vi "Current_Step.vi"   [LabVIEW 2019]
uses:
  Instrument_Setup.vi
  Global/Global Variables/Data_Display_global.vi
  Global/Global Variables/global.vi
  Equipment/Keithley 24XX/Keithley 24XX.lvlib
types:
  T1 = typedef "16T-Cluster.ctl" = cluster{"Clamp":bool, "Switch Heater":bool, "Go to Zero":bool, "Go to set":bool, "Go to Hold":bool, "Clamped":bool, "Quenched":bool, "Rate limit":bool, "Persistent":bool, "Hold":bool, "Set":bool, "Zero":bool, "Magnet (T)":dbl, "Leads (T)":dbl, "Magnet T (K)":dbl, "Switch":bool, "Setpoint (T)":dbl, "Rate (T/min)":dbl, "Select":bool, "Sweeping":bool}
  T2 = typedef "PSIO.ctl" = cluster{"Address":T3, "Version":enum16{"PS", "IPS"}}
  T3 = typedef "OxfordAddress.ctl" = cluster{"Com Port":i32, "ISOBUS Address":i32, "GPIB Address":i16, "Communication":enum16{"RS232", "ISOBUS", "GPIB", "Gateway"}}
  T4 = cluster{"Version\n":string, "Max Sweep(4.2K)":dbl[unit], "Max Sweep(2.2K)":dbl[unit], "Switch htr dly":dbl[unit], "Max Field(4.2K)":dbl[unit], "Max Field(2.2K)":dbl[unit], "Max lead res":dbl[unit], "IO Info":T2}
  T5 = typedef "15T-Cluster.ctl" = cluster{"Magnet (T)":dbl, "Leads (T)":dbl, "Setpoint (T)":dbl, "Rate (T/min)":dbl, "Set":bool, "Zero":bool, "Hold":bool, "Go to zero":bool, "Go to Hold":bool, "Go to Set":bool, "Clamp":bool, "Switch Heater":bool, "Rate limit":bool, "Switch":bool, "Clamped":bool, "Persistent":bool, "Quenched":bool, "Sweeping":bool, "Select":bool}
  T6 = cluster{"Version\n":string, "Max Sweep":dbl[unit], "Max Field":dbl[unit], "IO Info":T2, "Switch htr dly":dbl[unit]}
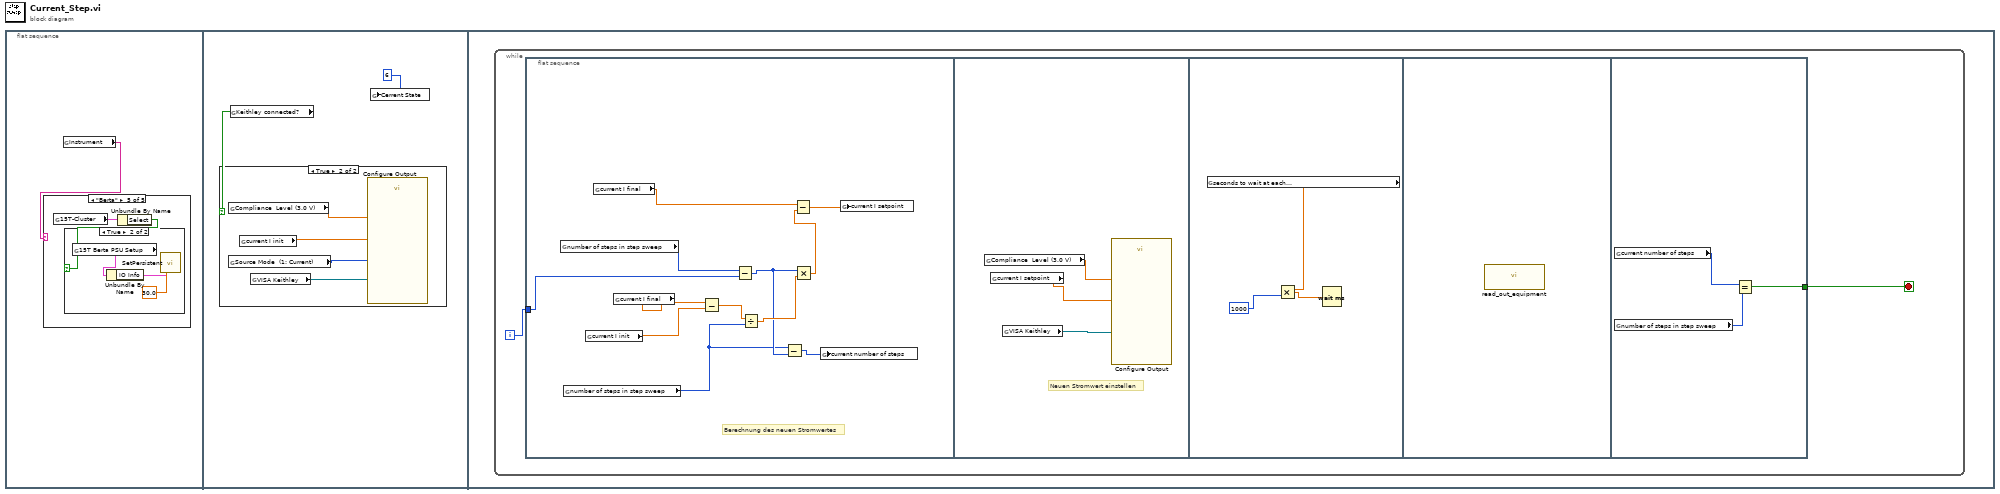
[diagram p0: block diagram]
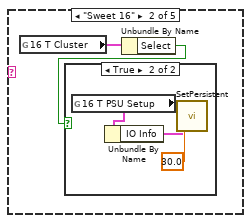
[diagram p3: hidden frame]
diagram:
  n1 = flat-sequence {
    frame #0 {
      n2 = global read "Instrument_Setup.vi" "Instrument"() -> (w1:string)
      n3 = case shown="\"Berta\"" w1 {
        frame "AMI", Default {
        }
        frame "Sweet 16" {
          n4 = global read "Data_Display_global.vi" "16 T Cluster"() -> (w3:T1)
          n5 = Unbundle By Name(w3) -> ("Select"=w2:bool)
          n6 = case shown="True" w2 {
            frame False {
            }
            frame True {
              n7 = global read "Instrument_Setup.vi" "16 T PSU Setup"() -> (w5:T4)
              n8 = Unbundle By Name(w5) -> ("IO Info"=w4:T2)
              n9 = call "SetPersistent.vi"("Switch Heater Dwell Time"=dbl[unit] 30.0, "IO Info"=w4) -> ()  [unwired: 1 in, 1 out]
            }
          }
        }
        frame "20T" {
        }
        frame "Mischer" {
        }
        frame "Berta" {
          n10 = global read "Data_Display_global.vi" "15T-Cluster"() -> (w8:T5)
          n11 = Unbundle By Name(w8) -> ("Select"=w7:bool)
          n12 = case shown="True" w7 {
            frame False {
            }
            frame True {
              n13 = global read "Instrument_Setup.vi" "15T Berta PSU Setup"() -> (w9:T6)
              n14 = Unbundle By Name(w9) -> ("IO Info"=w10:T2)
              n15 = call "SetPersistent.vi"("Switch Heater Dwell Time"=dbl[unit] 30.0, "IO Info"=w10) -> ()  [unwired: 1 in, 1 out]
            }
          }
        }
      }
    }
    frame #1 {
      n16 = global read "Instrument_Setup.vi" "Keithley connected?"() -> (w12:bool)
      n17 = case shown="True" w12 {
        frame False {
        }
        frame True {
          n18 = global read "Instrument_Setup.vi" "Compliance  Level (3.0 V)"() -> (w15:dbl)
          n19 = global read "Instrument_Setup.vi" "Source Mode  (1: Current)"() -> (w14:u16)
          n20 = global read "global.vi" "current I init"() -> (w16:dbl)
          n21 = global read "Instrument_Setup.vi" "VISA Keithley"() -> (w17:refnum<visa-resource-name>)
          n22 = call "Configure Output.vi"("Source Mode  (0: Voltage)"=w14, "Compliance  Level (3.0V)"=w15, "Output Level (0)"=w16, "VISA resource name"=w17) -> ()  [unwired: 6 in, 2 out]
        }
      }
      n23 = global write "global.vi" "Cerrent State"(6) -> ()
    }
    frame #2 {
      n24 = while {
        i -> [w18]
        stop <- w19 stop-if-true
        n25 = flat-sequence {
          tunnel: w18 -> [w27]
          tunnel: [w38] -> w19
          frame #0 {
            # "Berechnung des neuen Stromwertes"
            n26 = global read "global.vi" "number of steps in step sweep"() -> (w23:i32)
            n27 = global read "global.vi" "number of steps in step sweep"() -> (w20:i32)
            n28 = global read "global.vi" "current I init"() -> (w22:dbl)
            n29 = global read "global.vi" "current I final"() -> (w26:dbl)
            n30 = global read "global.vi" "current I final"() -> (w21:dbl)
            n31 = Subtract(x=w21, y=w22) -> (x-y=w28:dbl)
            n32 = Subtract(x=w23, y=w27) -> (x-y=w29:i32)
            n33 = Divide(x=w28, y=w20) -> (x/y=w30:dbl)
            n34 = Subtract(x=w20, y=w29) -> (x-y=w24:i32)
            n35 = Multiply(x=w29, y=w30) -> (x*y=w31:dbl)
            n36 = Subtract ("Subtrahieren")(x=w26, y=w31) -> (x-y=w25:dbl)
            n37 = global write "Data_Display_global.vi" "current number of steps"(w24) -> ()
            n38 = global write "Data_Display_global.vi" "current I setpoint"(w25) -> ()
          }
          frame #1 {
            # "Neuen Stromwert einstellen"
            n39 = global read "Instrument_Setup.vi" "Compliance  Level (3.0 V)"() -> (w32:dbl)
            n40 = global read "Data_Display_global.vi" "current I setpoint"() -> (w34:dbl)
            n41 = global read "Instrument_Setup.vi" "VISA Keithley"() -> (w33:refnum<visa-resource-name>)
            n42 = call "Configure Output.vi"("Compliance  Level (3.0V)"=w32, "Output Level (0)"=w34, "VISA resource name"=w33) -> ()  [unwired: 7 in, 2 out]
          }
          frame #2 {
            n43 = global read "Instrument_Setup.vi" "seconds to wait at each\ncurrent step in a I-step sweep"() -> (w37:dbl)
            n44 = Multiply(x=w37, y=u32 1000 ("milliseconds to wait")) -> (x*y=w35:dbl)
            n45 = Wait (ms)(milliseconds to wait=w35) -> ()  [unwired: 1 out]
          }
          frame #3 {
            n46 = call "read_out_equipment.vi"() -> ()  [unwired: 1 in]
          }
          frame #4 {
            n47 = global read "Data_Display_global.vi" "current number of steps"() -> (w39:i32)
            n48 = global read "global.vi" "number of steps in step sweep"() -> (w40:i32)
            n49 = Equal?(x=w39, y=w40) -> (x = y?=w38:bool)
          }
        }
      }
    }
  }
